vi "RIGOL DS1000 Series Acquire Continuous Waveform.vi"() -> ()   [LabVIEW 2012]
doc: "This example shows how to use autosetup and acquire a waveform on a single channel."
uses:
  Public/Data/Read (Single Waveform).vi
  <vilib>/measure/madcrms.llb/Basic Averaged DC-RMS for 1 Chan.vi
  RIGOL DS1000 Series.lvlib
  <vilib>/measure/NI_MAPro.lvlib
panel:
  out "IRMS":dbl
  out "VRMS":dbl
  in  "Channel (0: Channel 1) 2":u16(ring) items=["Channel 1", "Channel 2", "Channel 3", "Channel 4"]
  out "Waveform Data 2":waveform(dbl)(graph)
  in  "Stop 2":bool
  in  "Timeout (10000 ms) 2":u32=10000
  in  "VISA resource name 2":refnum<visa-resource-name>
  in  "Channel (0: Channel 1)":u16(ring) items=["Channel 1", "Channel 2", "Channel 3", "Channel 4"]
  in  "Stop":bool
  in  "Timeout (10000 ms)":u32=10000
  out "Waveform Data":waveform(dbl)(graph)
  in  "VISA resource name":refnum<visa-resource-name>
  # "(c) 2010-2012, RIGOL Technologies, Inc.  All Rights Reserved."
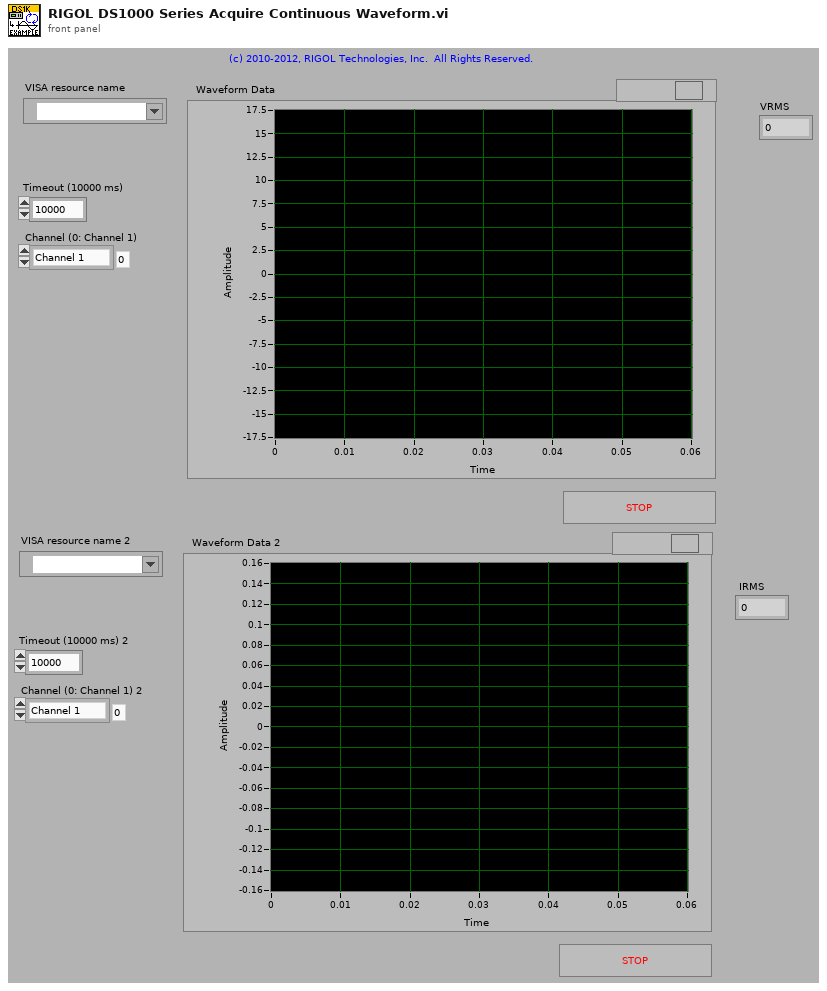
[diagram p1: front panel]
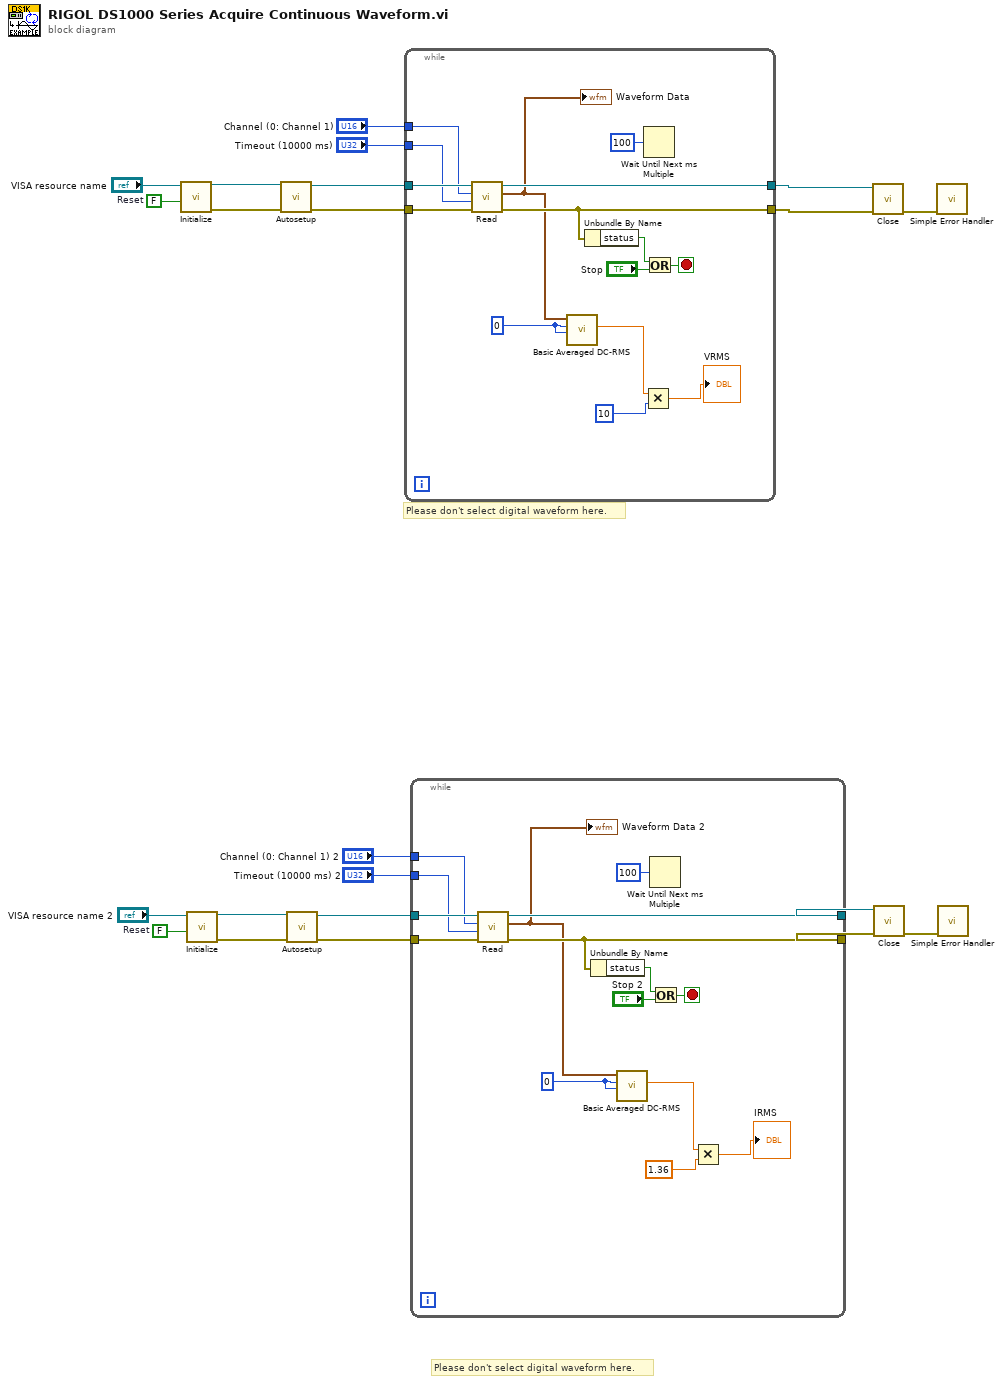
[diagram p0: block diagram]
diagram:
  w1 = FALSE  # Reset
  w12 = FALSE  # Reset
  # "Please don't select digital waveform here."
  # "Please don't select digital waveform here."
  n1 = call "Initialize.vi"("Reset (True)"=w12, "VISA resource name"="VISA resource name") -> ("error out"=w17:errorcluster, "VISA resource name out"=w16:refnum<visa-resource-name>)  [unwired: 2 in, 6 out]
  n2 = call "Initialize.vi"("Reset (True)"=w1, "VISA resource name"="VISA resource name 2") -> ("error out"=w6:errorcluster, "VISA resource name out"=w5:refnum<visa-resource-name>)  [unwired: 2 in, 6 out]
  n3 = call "Autosetup.vi"("error in (no error)"=w17, "VISA resource name"=w16) -> ("error out"=w14:errorcluster, "VISA resource name out"=w15:refnum<visa-resource-name>)  [unwired: 8 out]
  n4 = call "Autosetup.vi"("error in (no error)"=w6, "VISA resource name"=w5) -> ("error out"=w3:errorcluster, "VISA resource name out"=w4:refnum<visa-resource-name>)  [unwired: 8 out]
  n5 = while {
    tunnel: w15 -> [w37]
    tunnel: w14 -> [w36]
    tunnel: [w35] -> w21
    tunnel: [w32] -> w20
    tunnel: "Timeout (10000 ms)" -> [w28]
    tunnel: "Channel (0: Channel 1)" -> [w29]
    stop <- w33 stop-if-true
    w26 = 0
    n6 = call-poly "Read.vi"("error in (no error)"=w36, "Timeout (10000 ms)"=w28, "Channel (0: Channel 1)"=w29, "VISA resource name"=w37) -> ("error out"=w32:errorcluster, "Waveform Data"=w27:waveform(dbl), "VISA resource name out"=w35:refnum<visa-resource-name>)  [unwired: 5 out]
    "Waveform Data" <- w27
    n7 = call-poly <vilib>:"Basic Averaged DC-RMS.vi"("window"=w26, "averaging type"=w26, "signal in"=w27) -> ("RMS value"=w25:dbl)  [unwired: 5 in, 3 out]
    n8 = Unbundle By Name(w32) -> ("status"=w31:bool)
    n9 = Multiply(x=w25, y=10) -> (x*y=→"VRMS":dbl)
    n10 = Wait Until Next ms Multiple(millisecond multiple=u32 100) -> ()  [unwired: 1 out]
    n11 = Or(x=w31, y="Stop") -> (x .or. y?=w33:bool)
  }
  n12 = while {
    tunnel: w4 -> [w52]
    tunnel: w3 -> [w51]
    tunnel: [w50] -> w10
    tunnel: [w47] -> w9
    tunnel: "Timeout (10000 ms) 2" -> [w43]
    tunnel: "Channel (0: Channel 1) 2" -> [w44]
    stop <- w48 stop-if-true
    w39 = 0
    n13 = call-poly "Read.vi"("error in (no error)"=w51, "Timeout (10000 ms)"=w43, "Channel (0: Channel 1)"=w44, "VISA resource name"=w52) -> ("error out"=w47:errorcluster, "Waveform Data"=w38:waveform(dbl), "VISA resource name out"=w50:refnum<visa-resource-name>)  [unwired: 5 out]
    "Waveform Data 2" <- w38
    n14 = Unbundle By Name(w47) -> ("status"=w46:bool)
    n15 = call-poly <vilib>:"Basic Averaged DC-RMS.vi"("window"=w39, "averaging type"=w39, "signal in"=w38) -> ("RMS value"=w40:dbl)  [unwired: 5 in, 3 out]
    n16 = Wait Until Next ms Multiple(millisecond multiple=u32 100) -> ()  [unwired: 1 out]
    n17 = Or(x=w46, y="Stop 2") -> (x .or. y?=w48:bool)
    n18 = Multiply(x=w40, y=1.36) -> (x*y=→"IRMS":dbl)
  }
  n19 = call "Close.vi"("error in (no error)"=w20, "VISA resource name"=w21) -> ("error out"=w22:errorcluster)  [unwired: 9 out]
  n20 = call "Close.vi"("error in (no error)"=w9, "VISA resource name"=w10) -> ("error out"=w11:errorcluster)  [unwired: 9 out]
  n21 = call <vilib>:"Simple Error Handler.vi"("error in (no error)"=w22) -> ()  [unwired: 1 in, 8 out]
  n22 = call <vilib>:"Simple Error Handler.vi"("error in (no error)"=w11) -> ()  [unwired: 1 in, 8 out]
